vi "FindOwningAppFromPath.vi"(8 "error in (no error)":errorcluster, 11 "LVClass path":path) -> (0 "error out":errorcluster, 2 "owning applications":refnum<vi>[](array[refnum]), 3 "Qualified Name":string)   [LabVIEW 2019, in "BlueUtilityScripts.lvlib"]
uses:
  BlueUtilityScripts.lvlib
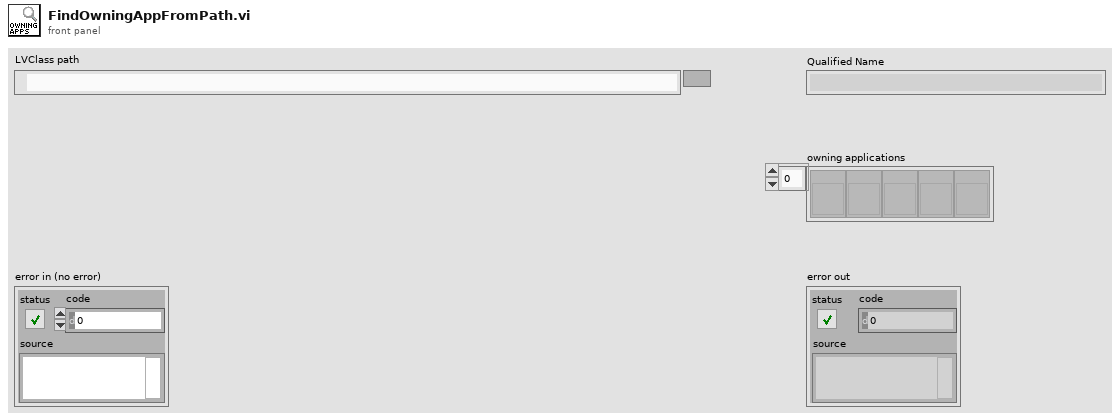
[diagram p1: front panel]
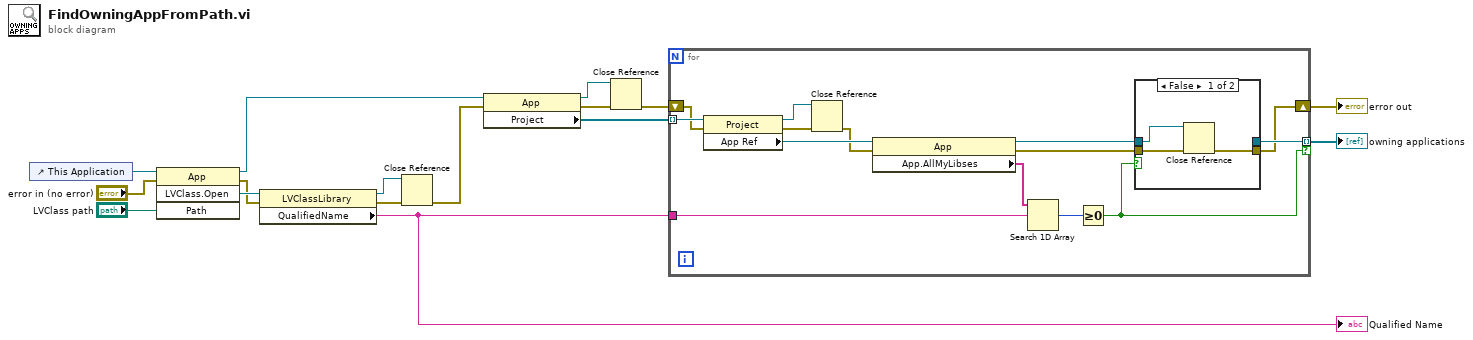
[diagram p0: block diagram]
diagram:
  n1 = control-ref of="This Application"() -> (w4:refnum<vi>)
  n2 = invoke class="App" method="LVClass.Open"(reference=w4, error in="error in (no error)", "Path"="LVClass path") -> (reference out=w5:refnum<vi>, error out=w6:errorcluster, "LVClass.Open"=w12:refnum<vi>)  [unwired: 1 in, 1 out]
  n3 = property class="LVClassLibrary"(reference=w12, error in=w6) -> (reference out=w11:refnum<vi>, error out=w10:errorcluster, "QualifiedName"=w8:string)
  "Qualified Name" <- w8
  n4 = Close Reference(reference=w11, error in (no error)=w10) -> (error out=w9:errorcluster)
  n5 = property class="App"(reference=w5, error in=w9) -> (reference out=w15:refnum<vi>, error out=w16:errorcluster, "Project"=w14:refnum<vi>[])
  n6 = Close Reference(reference=w15, error in (no error)=w16) -> (error out=w7:errorcluster)
  n7 = for {
    tunnel: w14 -> [w30] mode=indexing
    tunnel: w8 -> [w27]
    tunnel: [w24] -> w3 mode=indexing if=w17
    shift-right: [w18] -> w1
    shift-left: w7 -> [w23]
    n8 = property class="Project"(reference=w30, error in=w23) -> (reference out=w21:refnum<vi>, error out=w22:errorcluster, "App Ref"=w29:refnum<vi>)
    n9 = Close Reference(reference=w21, error in (no error)=w22) -> (error out=w20:errorcluster)
    n10 = property class="App"(reference=w29, error in=w20) -> (reference out=w25:refnum<vi>, error out=w19:errorcluster, "App.AllMyLibses"=w28:string[])
    n11 = Search 1D Array(1D array=w28, element=w27) -> (index of element=w26:i32)  [unwired: 1 in]
    n12 = Greater Or Equal To 0?(x=w26) -> (x >= 0?=w17:bool)
    n13 = case shown="False" w17 {
      tunnel: w25 -> [w33 w35]
      tunnel: [_ w35] -> w24
      tunnel: w19 -> [w32 w34]
      tunnel: [w31 w34] -> w18
      frame False {
        n14 = Close Reference(reference=w33, error in (no error)=w32) -> (error out=w31:errorcluster)
      }
      frame True {
      }
    }
  }
  "owning applications" <- w3
  "error out" <- w1
